vi "test.vi"(8 "error in (no error)":errorcluster, 11 "RSA in":refnum<class "RSA.lvclass">) -> (0 "error out":errorcluster, 3 "RSA out":refnum<class "RSA.lvclass">)   [LabVIEW 2012, in "RSA.lvclass"]
uses:
  RSA.lvclass
panel:
  out "actuator out":dbl
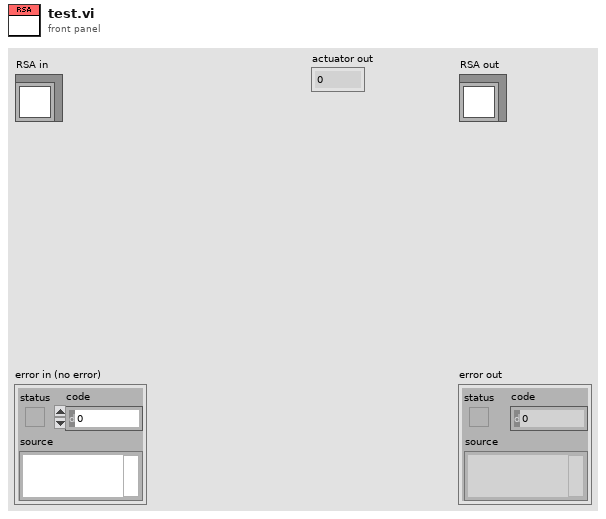
[diagram p1: front panel]
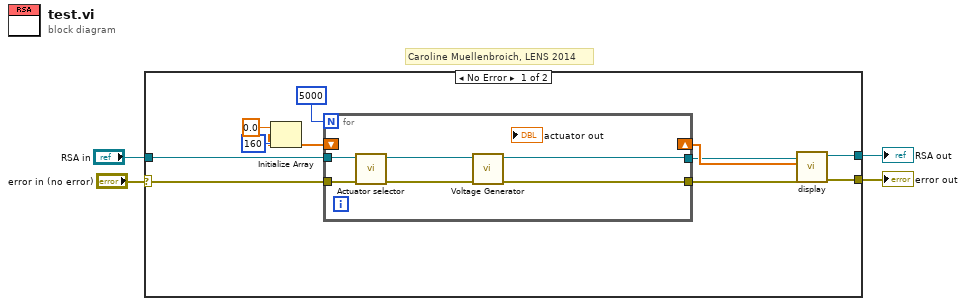
[diagram p0: block diagram]
diagram:
  # "Caroline Muellenbroich, LENS 2014"
  n1 = case shown="No Error" "error in (no error)" {
    selector: "error in (no error)" -> [w15 w22]
    tunnel: [w10 w23] -> w2
    tunnel: "RSA in" -> [w13 w23]
    tunnel: [w11 w22] -> w1
    frame No Error {
      n2 = Initialize Array(0.0 ("element"), 160 ("dimension size")) -> (w7:dbl[])
      n3 = for {
        N: 5000 -> [_]
        tunnel: w13 -> [w21]
        tunnel: w15 -> [w20]
        shift-right: [_] -> w12
        shift-left: w7 -> [_]
        tunnel: [w17] -> w6
        tunnel: [w16] -> w5
        n4 = call-dynamic "Actuator selector.vi"("error in (no error)"=w20, "RSA in"=w21) -> ("error out"=w18:errorcluster, "RSA out"=w19:refnum<class "RSA.lvclass">)  [unwired: 8 in]
        n5 = call "Voltage Generator.vi"("error in (no error)"=w18, "RSA in"=w19) -> ("error out"=w16:errorcluster, "RSA out"=w17:refnum<class "RSA.lvclass">)  [unwired: 8 in]
      }
      n6 = call-dynamic "display.vi"("error in (no error)"=w5, "current plus 1 in"=w12, "RSA in"=w6) -> ("error out"=w11:errorcluster, "RSA out"=w10:refnum<class "RSA.lvclass">)  [unwired: 7 in]
    }
    frame Error {
    }
  }
  "error out" <- w1
  "RSA out" <- w2
